vi "Autonomous Independent.vi"() -> ()   [LabVIEW 2015]
doc: "This VI is called when autonomous begins, and will automatically be terminated when autonomous ends. You can carry out timed or sensor driven robot movement independently without needing to return to the caller."
uses:
  <vilib>/Rock Robotics/WPI/Utilities/WPI_GetSetVariantRefNum.vi
  <vilib>/Rock Robotics/Network Tables/NT Read String.vi
  <vilib>/Rock Robotics/Network Tables/NT Write Number.vi
  <vilib>/addons/control/pid/pid.llb/PID (DBL).vi
  Robot Global Data.vi
  <vilib>/Rock Robotics/Network Tables/NT Write Numeric Array.vi
  <vilib>/addons/control/pid/NI_PID_pid.lvlib
  navX Library v2/navX Library v2.lvlib
panel:
  in  "Single Turn Gains":T1={"proportional gain (Kc)"=1.0, "integral time (Ti, min)"=0.01, "derivative time (Td, min)"=0.0} {"derivative time (Td, min)" format="%.3f"; "integral time (Ti, min)" format="%.3f"; "proportional gain (Kc)" format="%.3f"}
  in  "Yaw":T1={"proportional gain (Kc)"=1.0, "integral time (Ti, min)"=0.01, "derivative time (Td, min)"=0.0} {"derivative time (Td, min)" format="%.3f"; "integral time (Ti, min)" format="%.3f"; "proportional gain (Kc)" format="%.3f"}
  out "Right Motor Speed":dbl(graph)
  out "Left Motor Speed":dbl(graph)
  out "Right Motor":dbl(graph)
  out "Left Motor":dbl(graph)
  in  "Distance":dbl
  in  "Speed Gains 4":T1={"proportional gain (Kc)"=1.0, "integral time (Ti, min)"=0.01, "derivative time (Td, min)"=0.0} {"derivative time (Td, min)" format="%.3f"; "integral time (Ti, min)" format="%.3f"; "proportional gain (Kc)" format="%.3f"}
  out "E1 Dist 2":dbl
  out "E2 Dist 2":dbl
  out "nav X Yaw 2":dbl
  out "nav X Yaw":dbl
  out "E2 Dist":dbl
  out "E1 Dist":dbl
  in  "Yaw Gains":T1={"proportional gain (Kc)"=1.0, "integral time (Ti, min)"=0.01, "derivative time (Td, min)"=0.0} {"derivative time (Td, min)" format="%.3f"; "integral time (Ti, min)" format="%.3f"; "proportional gain (Kc)" format="%.3f"}
  # "Be sure to right-click and choose Data Operations>>Make Current Value default if you want to save the array values with the VI"
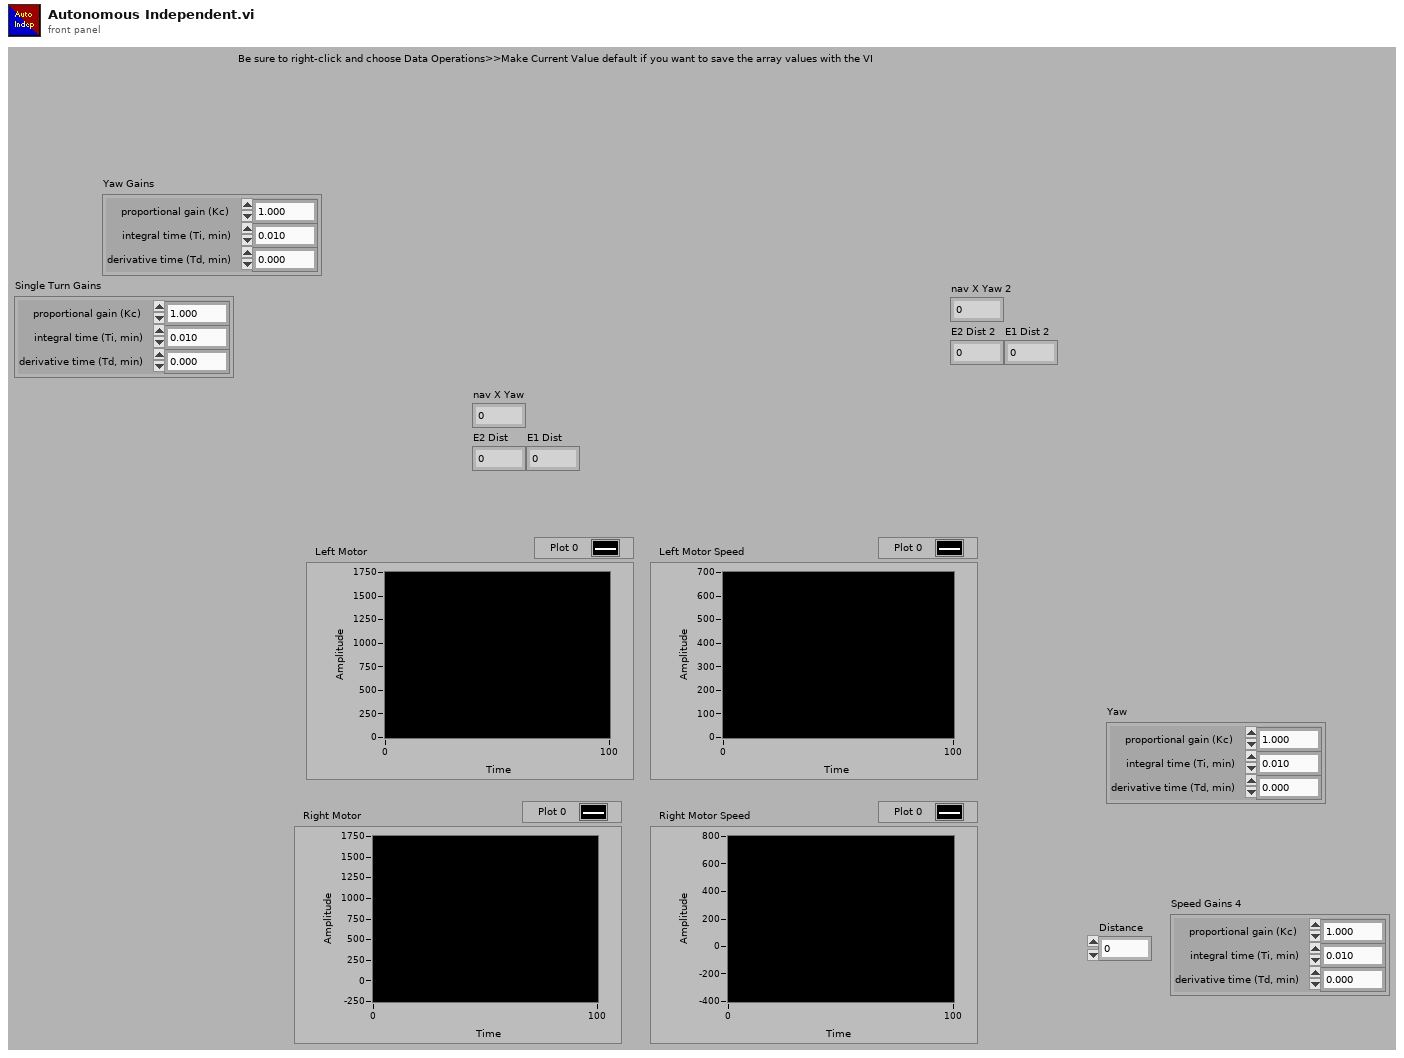
[diagram p1: front panel]
types:
  T1 = cluster{"proportional gain (Kc)":dbl, "integral time (Ti, min)":dbl, "derivative time (Td, min)":dbl}
  T2 = typedef "WPI_JoystickDevRef.ctl" = cluster{"Device":T3}
  T3 = typedef "WPI_JoystickDeviceEnum.ctl" = enum16{"USB 0", "USB 1", "USB 2", "USB 3", "USB 4", "USB 5"}
  T4 = typedef "navX Library v2.lvlib/Z900_navX_DeviceTypeDef.ctl" = cluster{"Interface":cluster{"Protocol":T5, "Update Rate (4Hz-60Hz)":u8, "navX Open TypeDef":variant}, "Notify Packet":refnum<notifier>, "Loop VI Refnum":refnum<vi>, "Ready to Close Occurrence Refnum":refnum<k4>}
  T5 = typedef "navX Library v2.lvlib/Z900_navX_ProtocolTypeDef.ctl" = enum16{"SERIAL", "I2C", "SPI"}
  T6 = typedef "WPI_EncoderDevRef.ctl" = cluster{"DevStatus":errorcluster, "EncoderIndex":T7, "CounterIndex":T8, "DistancePerCount":dbl, "Decoding Type":T9}
  T7 = typedef "FPGA_EncoderIdx.ctl" = enum8{"Enc 0", "Enc 1", "Enc 2", "Enc 3", "Enc 4", "Enc 5", "Enc 6", "Enc 7", "Invalid"}
  T8 = typedef "FPGA_CounterCtrSystemIndex.ctl" = enum8{"Ctr 0", "Ctr 1", "Ctr 2", "Ctr 3", "Ctr 4", "Ctr 5", "Ctr 6", "Ctr 7", "Invalid"}
  T9 = typedef "WPI_EncoderType.ctl" = enum16{"1x", "2x", "4x"}
  T10 = cluster{"Yaw":dbl, "Roll":dbl, "Pitch":dbl, "Heading":dbl, "Fused Heading":dbl}
  T11 = typedef "WPI_RobotDriveDevRef.ctl" = cluster{"DevStatus":errorcluster, "Motors[]":T12[], "Square Inputs":bool, "Max Output":dbl}
  T12 = typedef "WPI_MotorControlDeviceRef.ctl" = cluster{"DeviceStatus":errorcluster, "Type":T13, "PWM":cluster{"PWM Channel":T14, "DeadBand":T15}, "CAN":cluster{"Device Number":u8, "Control Mode":T16, "Semaphore":T17, "Max Vout":dbl, "TalonSRX Control Mode":T18}, "Invert":bool}
  T13 = typedef "WPI_MotorControlType.ctl" = enum16{"PWM", "CAN", "CANTalonSRX"}
  T14 = typedef "FPGA_DIOPWMChannel.ctl" = enum8{"PWM 0", "PWM 1", "PWM 2", "PWM 3", "PWM 4", "PWM 5", "PWM 6", "PWM 7", "PWM 8", "PWM 9", "PWM MXP 0", "PWM MXP 1", "PWM MXP 2", "PWM MXP 3", "PWM MXP 4", "PWM MXP 5", "PWM MXP 6", "PWM MXP 7", "PWM MXP 8", "PWM MXP 9", "Invalid"}
  T15 = typedef "WPI_PWMDeadband.ctl" = cluster{"Name":string, "maxPositivePwm":i32, "minPositivePwm":i32, "centerPwm":i32, "maxNegativePwm":i32, "minNegativePwm":i32, "angularRange":u16}
  T16 = typedef "WPI_CANJaguar_ControlMode.ctl" = enum8{"Percent VBus", "Current", "Speed", "Position", "Voltage"}
  T17 = typedef "Semaphore RefNum" = refnum<k1>
  T18 = typedef "WPI_CANTalonSRX_APIControlMode.ctl" = enum8{"Percent VBus", "Speed", "Position", "Slave", "Unchanged / Invalid", "Voltage Compensation", "Current", "Motion Profile"}
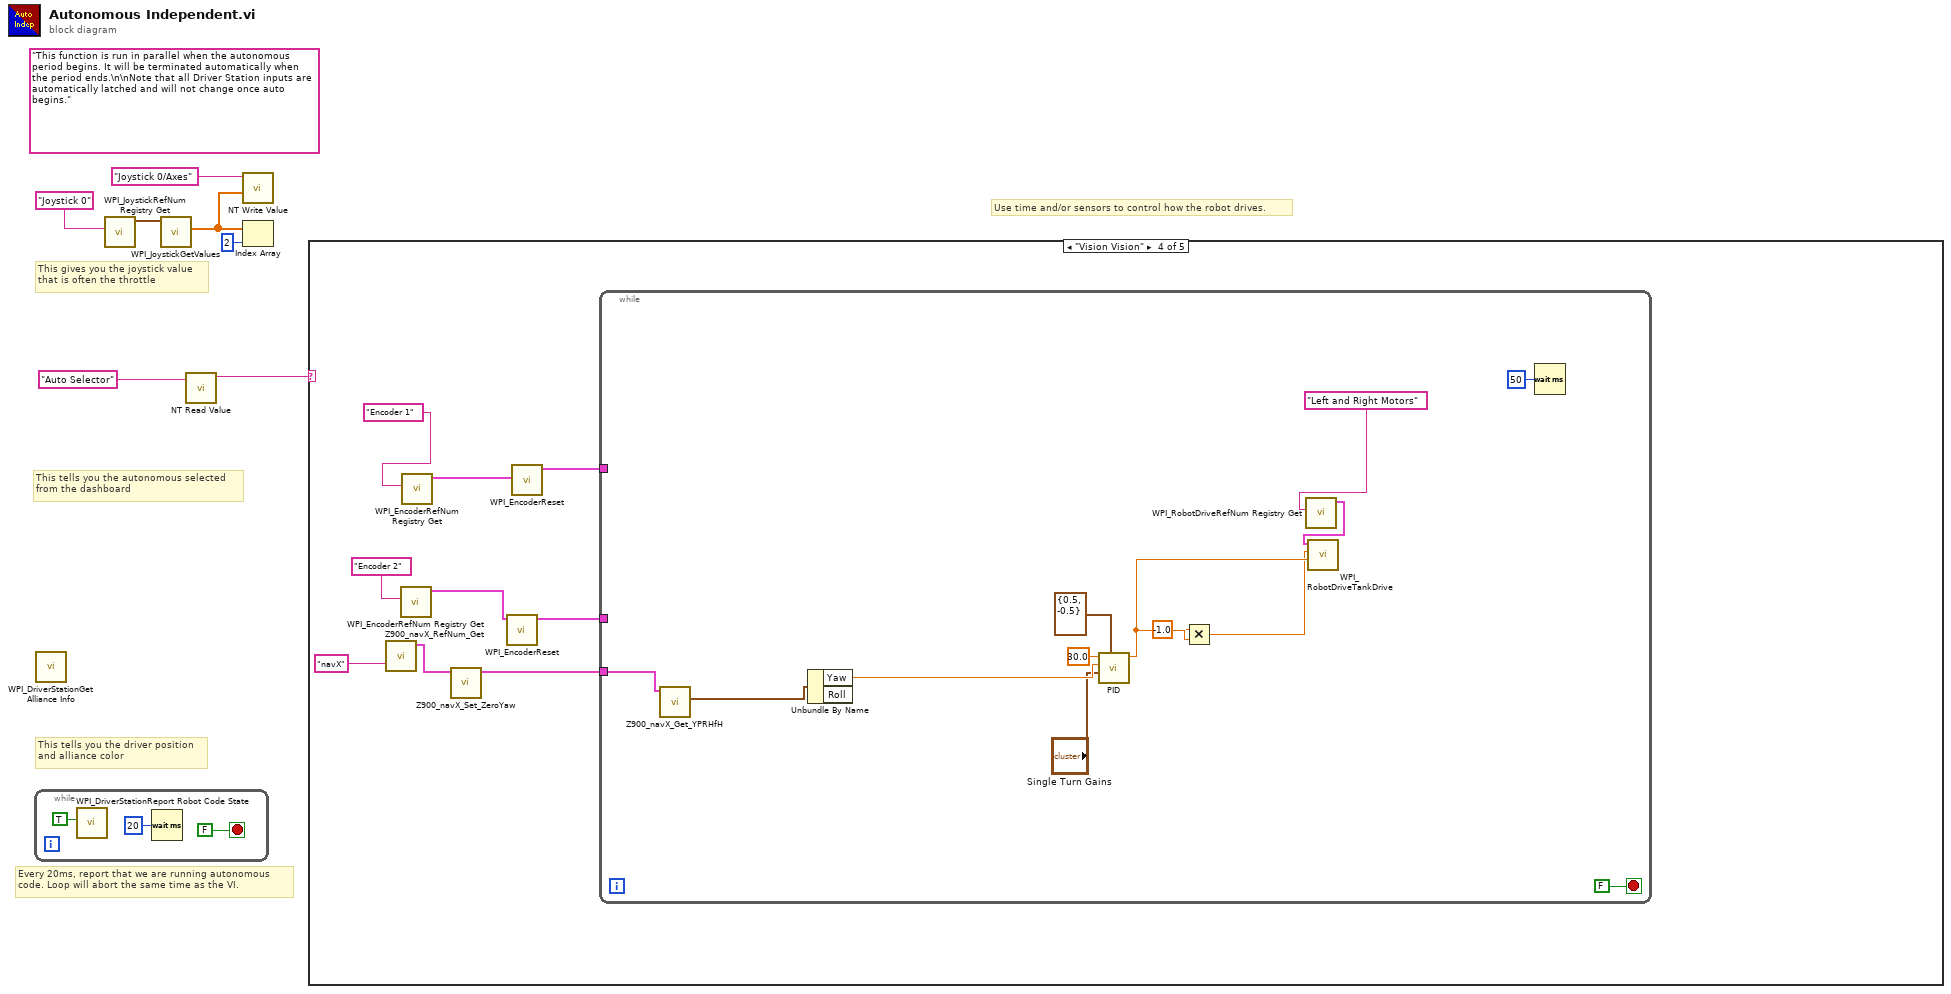
[diagram p0: block diagram]
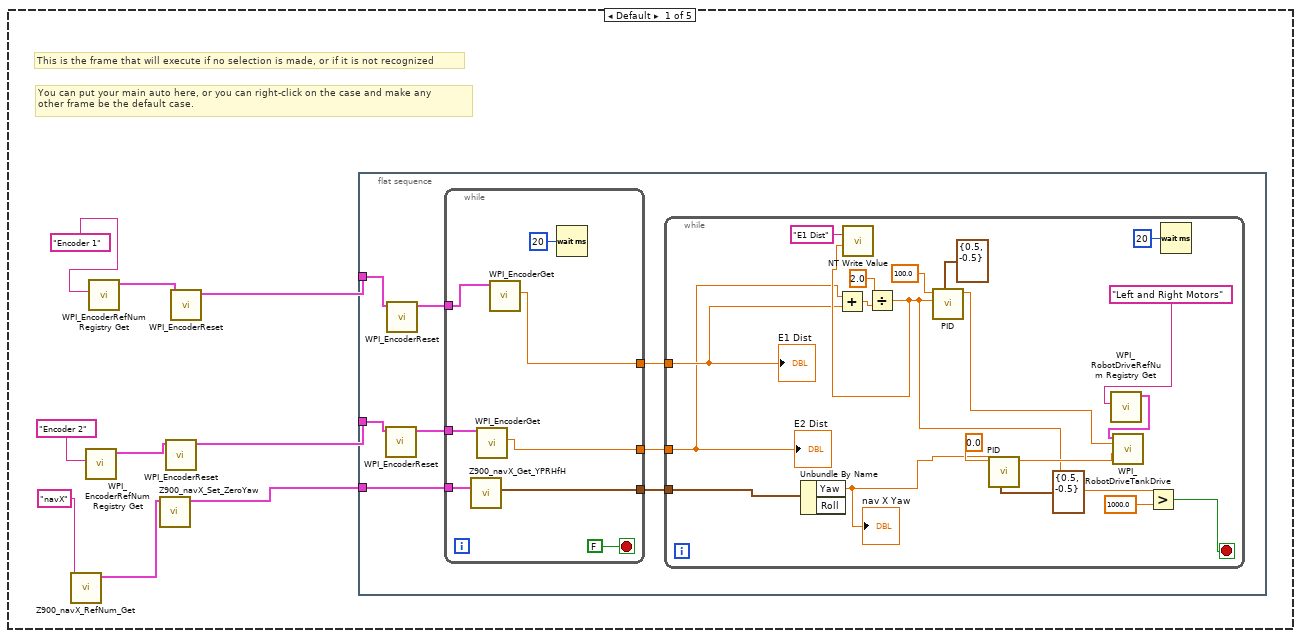
[diagram p2: hidden frame]
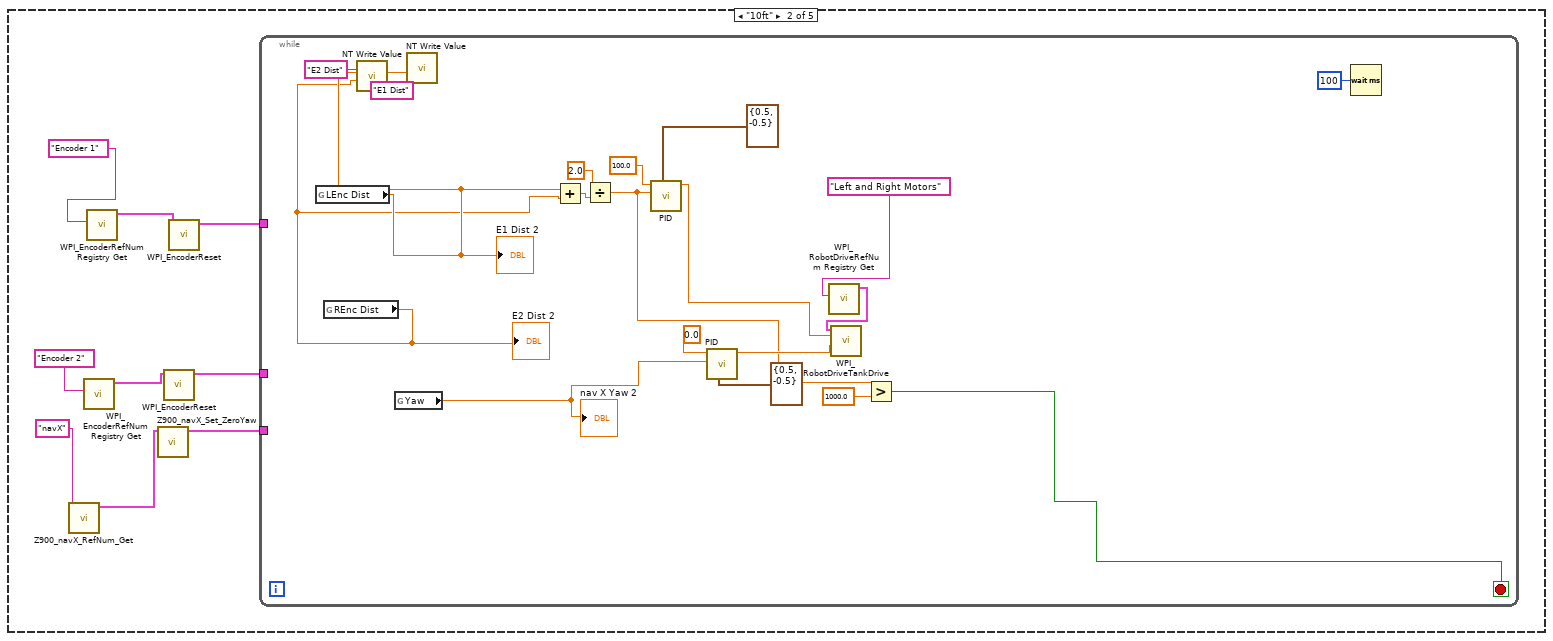
[diagram p3: hidden frame]
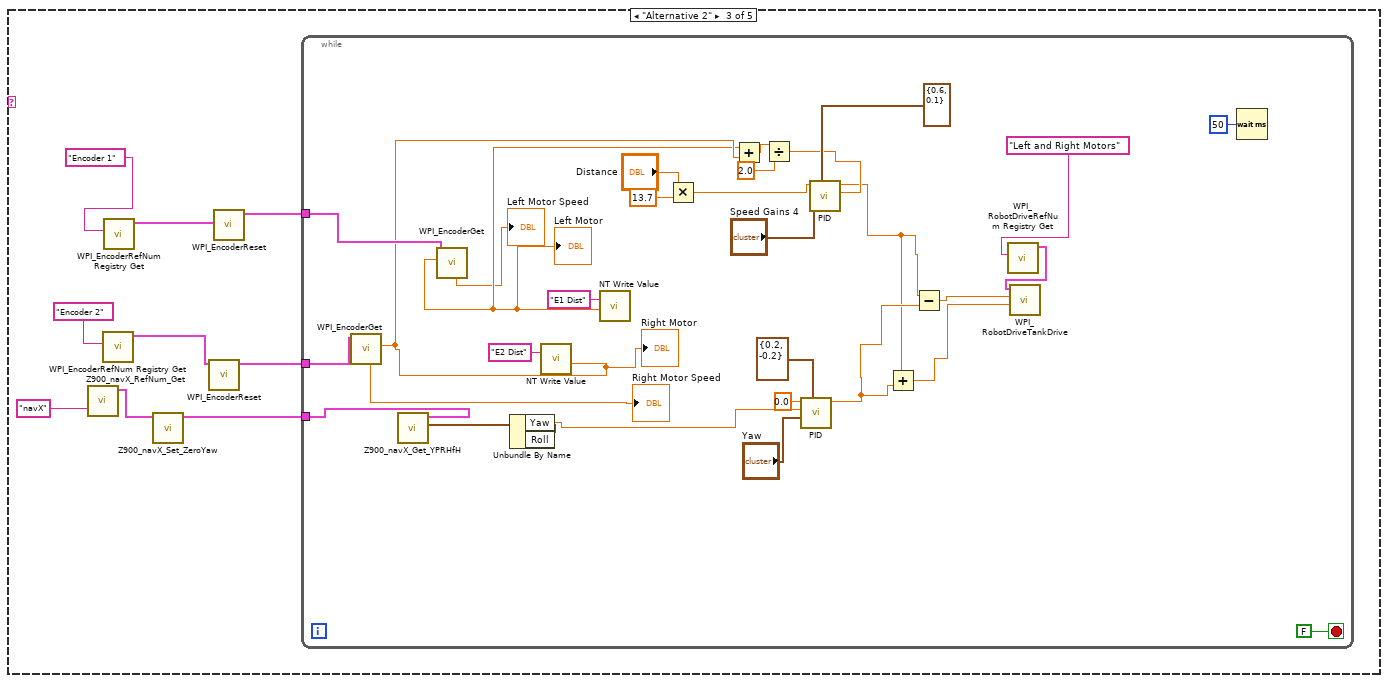
[diagram p4: hidden frame]
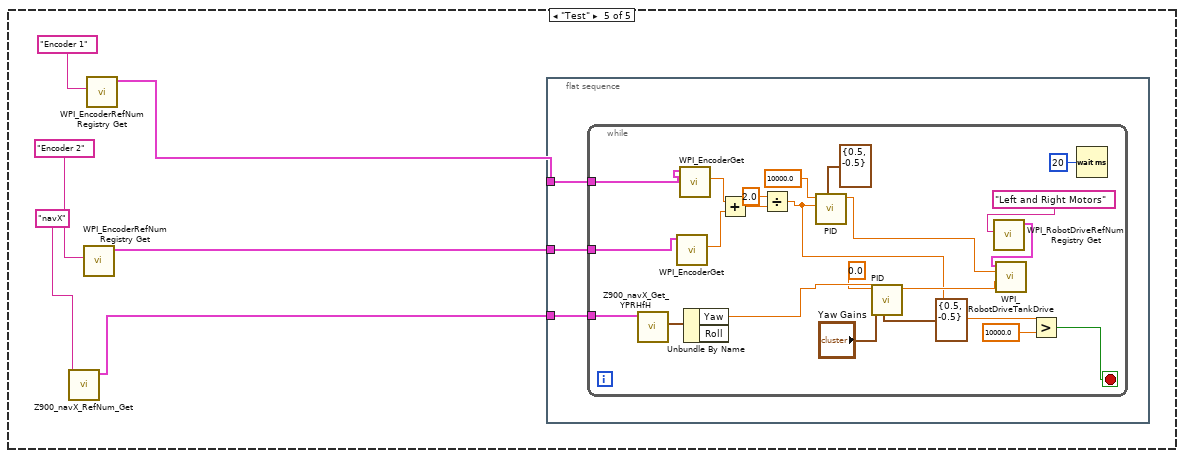
[diagram p5: hidden frame]
diagram:
  (unwired) "This function is run in parallel when the autonomous period begins. It will be terminated automatically when the period ends.\n\nNote that all Driver Station inputs are automatically latched and will not change once auto begins."
  # "This tells you the autonomous selected\nfrom the dashboard"
  # "Every 20ms, report that we are running autonomous\ncode. Loop will abort the same time as the VI."
  # "This gives you the joystick value\nthat is often the throttle"
  # "Use time and/or sensors to control how the robot drives."
  # "This tells you the driver position\nand alliance color"
  n1 = while {
    stop <- FALSE stop-if-true
    n2 = call <vilib>:"WPI_DriverStationReport Robot Code State.vi"("Autonomous"=TRUE) -> ()  [unwired: 10 in, 1 out]
    n3 = Wait (ms)(milliseconds to wait=u32 20) -> ()  [unwired: 1 out]
  }
  n4 = call <vilib>:"WPI_DriverStationGet Alliance Info.vi"() -> ()  [unwired: 12 out]
  n5 = call <vilib>:"WPI_JoystickRefNum Registry Get.vi"("refnum name"="Joystick 0") -> ("JoystickDevRef"=w6:T2)  [unwired: 1 in, 9 out]
  n6 = call <vilib>:"WPI_JoystickGetValues.vi"("JoystickDevRef"=w6) -> ("Axes"=w2:dbl[])  [unwired: 6 in, 4 out]
  n7 = call-poly <vilib>:"NT Read Value.vi"("Name"="Auto Selector") -> ("String"=w3:string)  [unwired: 9 in, 1 out]
  n8 = call-poly <vilib>:"NT Write Value.vi"("Numeric Array"=w2, "Name"="Joystick 0/Axes") -> ()  [unwired: 9 in, 1 out]
  n9 = Index Array(array=w2, index=2) -> ()  [unwired: 1 out]
  n10 = case shown="\"Vision Vision\"" w3 {
    frame Default {
      # "You can put your main auto here, or you can right-click on the case and make any\nother frame be the default case."
      # "This is the frame that will execute if no selection is made, or if it is not recognized"
      n11 = call "Z900_navX_RefNum_Get.vi"("refnum name"="navX") -> ("navX Device"=w13:T4)  [unwired: 9 in, 1 out]
      n12 = call <vilib>:"WPI_EncoderRefNum Registry Get.vi"("refnum name"="Encoder 2") -> ("EncoderDevRef"=w15:T6)  [unwired: 9 in, 1 out]
      n13 = call <vilib>:"WPI_EncoderRefNum Registry Get.vi"("refnum name"="Encoder 1") -> ("EncoderDevRef"=w17:T6)  [unwired: 9 in, 1 out]
      n14 = call "Z900_navX_Set_ZeroYaw.vi"("navX Device"=w13) -> ("navX Device"=w12:T4)  [unwired: 9 in, 1 out]
      n15 = call <vilib>:"WPI_EncoderReset.vi"("EncoderDevRef"=w15) -> ("EncoderDevRef"=w14:T6)  [unwired: 9 in, 1 out]
      n16 = call <vilib>:"WPI_EncoderReset.vi"("EncoderDevRef"=w17) -> ("EncoderDevRef"=w16:T6)  [unwired: 9 in, 1 out]
      n17 = flat-sequence {
        tunnel: w16 -> [w27]
        tunnel: w14 -> [w26]
        tunnel: w12 -> [w25]
        frame #0 {
          n18 = call <vilib>:"WPI_EncoderReset.vi"("EncoderDevRef"=w26) -> ("EncoderDevRef"=w24:T6)  [unwired: 9 in, 1 out]
          n19 = call <vilib>:"WPI_EncoderReset.vi"("EncoderDevRef"=w27) -> ("EncoderDevRef"=w23:T6)  [unwired: 9 in, 1 out]
          n20 = while {
            tunnel: w25 -> [w32]
            tunnel: w24 -> [w33]
            tunnel: w23 -> [w34]
            tunnel: [w31] -> w22
            tunnel: [w30] -> w21
            tunnel: [w29] -> w20
            stop <- FALSE stop-if-true
            n21 = call "Z900_navX_Get_YPRHfH.vi"("navX Device"=w32) -> ("YRPHfH"=w31:T10)  [unwired: 7 in, 3 out]
            n22 = call <vilib>:"WPI_EncoderGet.vi"("EncoderDevRef"=w33) -> ("Distance"=w30:dbl)  [unwired: 5 in, 5 out]
            n23 = call <vilib>:"WPI_EncoderGet.vi"("EncoderDevRef"=w34) -> ("Distance"=w29:dbl)  [unwired: 5 in, 5 out]
            n24 = Wait (ms)(milliseconds to wait=u32 20) -> ()  [unwired: 1 out]
          }
          n25 = while {
            tunnel: w22 -> [w39]
            tunnel: w21 -> [w37]
            tunnel: w20 -> [w38]
            stop <- w43 stop-if-true
            n26 = Unbundle By Name(w39) -> ("Yaw"=w40:dbl)  [unwired: 1 out]
            "nav X Yaw" <- w40
            n27 = Add(x=w37, y=w38) -> (x+y=w54:dbl)
            n28 = Divide(x=2.0, y=w54) -> (x/y=w42:dbl)
            n29 = call-poly <vilib>:"NT Write Value.vi"("Numeric"=w42, "Name"="E1 Dist") -> ()  [unwired: 9 in, 1 out]
            n30 = call-poly <vilib>:"PID.vi"("output range"=cluster{"output high":dbl, "output low":dbl} {"output high"=0.5, "output low"=-0.5}, "process variable"=w42, "setpoint"=100.0) -> ("output"=w47:dbl)  [unwired: 7 in, 1 out]
            n31 = call-poly <vilib>:"PID.vi"("output range"=cluster{"output high":dbl, "output low":dbl} {"output high"=0.5, "output low"=-0.5}, "process variable"=w40, "setpoint"=0.0) -> ("output"=w46:dbl)  [unwired: 7 in, 1 out]
            n32 = call <vilib>:"WPI_RobotDriveRefNum Registry Get.vi"("refnum name"="Left and Right Motors") -> ("RobotDriveDevRef"=w49:T11)  [unwired: 9 in, 1 out]
            n33 = call <vilib>:"WPI_RobotDriveTankDrive.vi"("Right axis value"=w46, "Left axis value"=w47, "RobotDriveDevRef"=w49) -> ()  [unwired: 6 in, 3 out]
            n34 = Greater?(x=w42, y=1000.0) -> (0:w43:bool)
            n35 = Wait (ms)(milliseconds to wait=u32 20) -> ()  [unwired: 1 out]
            "E2 Dist" <- w37
            "E1 Dist" <- w38
          }
        }
      }
    }
    frame "10ft" {
      n36 = call "Z900_navX_RefNum_Get.vi"("refnum name"="navX") -> ("navX Device"=w57:T4)  [unwired: 9 in, 1 out]
      n37 = call <vilib>:"WPI_EncoderRefNum Registry Get.vi"("refnum name"="Encoder 2") -> ("EncoderDevRef"=w59:T6)  [unwired: 9 in, 1 out]
      n38 = call <vilib>:"WPI_EncoderRefNum Registry Get.vi"("refnum name"="Encoder 1") -> ("EncoderDevRef"=w61:T6)  [unwired: 9 in, 1 out]
      n39 = call "Z900_navX_Set_ZeroYaw.vi"("navX Device"=w57) -> ("navX Device"=w56:T4)  [unwired: 9 in, 1 out]
      n40 = call <vilib>:"WPI_EncoderReset.vi"("EncoderDevRef"=w59) -> ("EncoderDevRef"=w58:T6)  [unwired: 9 in, 1 out]
      n41 = call <vilib>:"WPI_EncoderReset.vi"("EncoderDevRef"=w61) -> ("EncoderDevRef"=w60:T6)  [unwired: 9 in, 1 out]
      n42 = while {
        tunnel: w60 -> [_]
        tunnel: w58 -> [_]
        tunnel: w56 -> [_]
        stop <- w64 stop-if-true
        n43 = global read "Robot Global Data.vi" "LEnc Dist"() -> (w67:dbl)
        "E1 Dist 2" <- w67
        n44 = global read "Robot Global Data.vi" "REnc Dist"() -> (w66:dbl)
        "E2 Dist 2" <- w66
        n45 = call-poly <vilib>:"NT Write Value.vi"("Numeric"=w66, "Name"="E2 Dist") -> ()  [unwired: 9 in, 1 out]
        n46 = global read "Robot Global Data.vi" "Yaw"() -> (w65:dbl)
        "nav X Yaw 2" <- w65
        n47 = call-poly <vilib>:"NT Write Value.vi"("Numeric"=w67, "Name"="E1 Dist") -> ()  [unwired: 9 in, 1 out]
        n48 = Add(x=w67, y=w66) -> (x+y=w81:dbl)
        n49 = Divide(x=2.0, y=w81) -> (x/y=w71:dbl)
        n50 = call-poly <vilib>:"PID.vi"("output range"=cluster{"output high":dbl, "output low":dbl} {"output high"=0.5, "output low"=-0.5}, "process variable"=w71, "setpoint"=100.0) -> ("output"=w75:dbl)  [unwired: 7 in, 1 out]
        n51 = call-poly <vilib>:"PID.vi"("output range"=cluster{"output high":dbl, "output low":dbl} {"output high"=0.5, "output low"=-0.5}, "process variable"=w65, "setpoint"=0.0) -> ("output"=w74:dbl)  [unwired: 7 in, 1 out]
        n52 = call <vilib>:"WPI_RobotDriveRefNum Registry Get.vi"("refnum name"="Left and Right Motors") -> ("RobotDriveDevRef"=w77:T11)  [unwired: 9 in, 1 out]
        n53 = call <vilib>:"WPI_RobotDriveTankDrive.vi"("Right axis value"=w74, "Left axis value"=w75, "RobotDriveDevRef"=w77) -> ()  [unwired: 6 in, 3 out]
        n54 = Greater?(x=w71, y=1000.0) -> (0:w64:bool)
        n55 = Wait (ms)(milliseconds to wait=u32 100) -> ()  [unwired: 1 out]
      }
    }
    frame "Alternative 2" {
      n56 = call "Z900_navX_RefNum_Get.vi"("refnum name"="navX") -> ("navX Device"=w84:T4)  [unwired: 9 in, 1 out]
      n57 = call <vilib>:"WPI_EncoderRefNum Registry Get.vi"("refnum name"="Encoder 2") -> ("EncoderDevRef"=w86:T6)  [unwired: 9 in, 1 out]
      n58 = call <vilib>:"WPI_EncoderRefNum Registry Get.vi"("refnum name"="Encoder 1") -> ("EncoderDevRef"=w88:T6)  [unwired: 9 in, 1 out]
      n59 = call "Z900_navX_Set_ZeroYaw.vi"("navX Device"=w84) -> ("navX Device"=w83:T4)  [unwired: 9 in, 1 out]
      n60 = call <vilib>:"WPI_EncoderReset.vi"("EncoderDevRef"=w86) -> ("EncoderDevRef"=w85:T6)  [unwired: 9 in, 1 out]
      n61 = call <vilib>:"WPI_EncoderReset.vi"("EncoderDevRef"=w88) -> ("EncoderDevRef"=w87:T6)  [unwired: 9 in, 1 out]
      n62 = while {
        tunnel: w87 -> [w114]
        tunnel: w85 -> [w113]
        tunnel: w83 -> [w112]
        stop <- FALSE stop-if-true
        n63 = call <vilib>:"WPI_EncoderGet.vi"("EncoderDevRef"=w113) -> ("Distance"=w103:dbl, "Rate"=→"Right Motor Speed":dbl)  [unwired: 5 in, 4 out]
        "Right Motor" <- w103
        n64 = call "Z900_navX_Get_YPRHfH.vi"("navX Device"=w112) -> ("YRPHfH"=w115:T10)  [unwired: 7 in, 3 out]
        n65 = call <vilib>:"WPI_EncoderGet.vi"("EncoderDevRef"=w114) -> ("Distance"=w102:dbl, "Rate"=→"Left Motor Speed":dbl)  [unwired: 5 in, 4 out]
        "Left Motor" <- w102
        n66 = Unbundle By Name(w115) -> ("Yaw"=w99:dbl)  [unwired: 1 out]
        n67 = call-poly <vilib>:"NT Write Value.vi"("Numeric"=w103, "Name"="E2 Dist") -> ()  [unwired: 9 in, 1 out]
        n68 = call-poly <vilib>:"NT Write Value.vi"("Numeric"=w102, "Name"="E1 Dist") -> ()  [unwired: 9 in, 1 out]
        n69 = Multiply(x="Distance", y=13.7) -> (x*y=w104:dbl)
        n70 = Add(x=w102, y=w103) -> (x+y=w109:dbl)
        n71 = Divide(x=w109, y=2.0) -> (x/y=w107:dbl)
        n72 = call-poly <vilib>:"PID.vi"("output range"=cluster{"output high":dbl, "output low":dbl} {"output high"=0.2, "output low"=-0.2}, "PID gains"="Yaw", "process variable"=w99, "setpoint"=0.0) -> ("output"=w97:dbl)  [unwired: 6 in, 1 out]
        n73 = call-poly <vilib>:"PID.vi"("output range"=cluster{"output high":dbl, "output low":dbl} {"output high"=0.6, "output low"=0.1}, "PID gains"="Speed Gains 4", "process variable"=w107, "setpoint"=w104) -> ("output"=w94:dbl)  [unwired: 6 in, 1 out]
        n74 = Add(x=w94, y=w97) -> (x+y=w96:dbl)
        n75 = Subtract(x=w94, y=w97) -> (x-y=w95:dbl)
        n76 = call <vilib>:"WPI_RobotDriveRefNum Registry Get.vi"("refnum name"="Left and Right Motors") -> ("RobotDriveDevRef"=w117:T11)  [unwired: 9 in, 1 out]
        n77 = call <vilib>:"WPI_RobotDriveTankDrive.vi"("Right axis value"=w96, "Left axis value"=w95, "RobotDriveDevRef"=w117) -> ()  [unwired: 6 in, 3 out]
        n78 = Wait (ms)(milliseconds to wait=u32 50) -> ()  [unwired: 1 out]
      }
    }
    frame "Vision Vision" {
      n79 = call "Z900_navX_RefNum_Get.vi"("refnum name"="navX") -> ("navX Device"=w123:T4)  [unwired: 9 in, 1 out]
      n80 = call <vilib>:"WPI_EncoderRefNum Registry Get.vi"("refnum name"="Encoder 2") -> ("EncoderDevRef"=w125:T6)  [unwired: 9 in, 1 out]
      n81 = call <vilib>:"WPI_EncoderRefNum Registry Get.vi"("refnum name"="Encoder 1") -> ("EncoderDevRef"=w127:T6)  [unwired: 9 in, 1 out]
      n82 = call "Z900_navX_Set_ZeroYaw.vi"("navX Device"=w123) -> ("navX Device"=w122:T4)  [unwired: 9 in, 1 out]
      n83 = call <vilib>:"WPI_EncoderReset.vi"("EncoderDevRef"=w125) -> ("EncoderDevRef"=w124:T6)  [unwired: 9 in, 1 out]
      n84 = call <vilib>:"WPI_EncoderReset.vi"("EncoderDevRef"=w127) -> ("EncoderDevRef"=w126:T6)  [unwired: 9 in, 1 out]
      n85 = while {
        tunnel: w126 -> [_]
        tunnel: w124 -> [_]
        tunnel: w122 -> [w137]
        stop <- FALSE stop-if-true
        n86 = call "Z900_navX_Get_YPRHfH.vi"("navX Device"=w137) -> ("YRPHfH"=w136:T10)  [unwired: 7 in, 3 out]
        n87 = Unbundle By Name(w136) -> ("Yaw"=w135:dbl)  [unwired: 1 out]
        n88 = call-poly <vilib>:"PID.vi"("output range"=cluster{"output high":dbl, "output low":dbl} {"output high"=0.5, "output low"=-0.5}, "PID gains"="Single Turn Gains", "process variable"=w135, "setpoint"=30.0) -> ("output"=w133:dbl)  [unwired: 6 in, 1 out]
        n89 = Multiply(x=-1.0, y=w133) -> (x*y=w131:dbl)
        n90 = call <vilib>:"WPI_RobotDriveRefNum Registry Get.vi"("refnum name"="Left and Right Motors") -> ("RobotDriveDevRef"=w142:T11)  [unwired: 9 in, 1 out]
        n91 = call <vilib>:"WPI_RobotDriveTankDrive.vi"("Right axis value"=w133, "Left axis value"=w131, "RobotDriveDevRef"=w142) -> ()  [unwired: 6 in, 3 out]
        n92 = Wait (ms)(milliseconds to wait=u32 50) -> ()  [unwired: 1 out]
      }
    }
    frame "Test" {
      n93 = call "Z900_navX_RefNum_Get.vi"("refnum name"="navX") -> ("navX Device"=w144:T4)  [unwired: 9 in, 1 out]
      n94 = call <vilib>:"WPI_EncoderRefNum Registry Get.vi"("refnum name"="Encoder 2") -> ("EncoderDevRef"=w145:T6)  [unwired: 9 in, 1 out]
      n95 = call <vilib>:"WPI_EncoderRefNum Registry Get.vi"("refnum name"="Encoder 1") -> ("EncoderDevRef"=w146:T6)  [unwired: 9 in, 1 out]
      n96 = flat-sequence {
        tunnel: w146 -> [w152]
        tunnel: w145 -> [w151]
        tunnel: w144 -> [w150]
        frame #0 {
          n97 = while {
            tunnel: w152 -> [w173]
            tunnel: w151 -> [w172]
            tunnel: w150 -> [w163]
            stop <- w153 stop-if-true
            n98 = call "Z900_navX_Get_YPRHfH.vi"("navX Device"=w163) -> ("YRPHfH"=w174:T10)  [unwired: 7 in, 3 out]
            n99 = call <vilib>:"WPI_EncoderGet.vi"("EncoderDevRef"=w172) -> ("Distance"=w169:dbl)  [unwired: 5 in, 5 out]
            n100 = call <vilib>:"WPI_EncoderGet.vi"("EncoderDevRef"=w173) -> ("Distance"=w170:dbl)  [unwired: 5 in, 5 out]
            n101 = Unbundle By Name(w174) -> ("Yaw"=w165:dbl)  [unwired: 1 out]
            n102 = Add(x=w170, y=w169) -> (x+y=w168:dbl)
            n103 = Divide(x=2.0, y=w168) -> (x/y=w155:dbl)
            n104 = call-poly <vilib>:"PID.vi"("output range"=cluster{"output high":dbl, "output low":dbl} {"output high"=0.5, "output low"=-0.5}, "process variable"=w155, "setpoint"=10000.0) -> ("output"=w159:dbl)  [unwired: 7 in, 1 out]
            n105 = call-poly <vilib>:"PID.vi"("output range"=cluster{"output high":dbl, "output low":dbl} {"output high"=0.5, "output low"=-0.5}, "PID gains"="Yaw Gains", "process variable"=w165, "setpoint"=0.0) -> ("output"=w158:dbl)  [unwired: 6 in, 1 out]
            n106 = call <vilib>:"WPI_RobotDriveRefNum Registry Get.vi"("refnum name"="Left and Right Motors") -> ("RobotDriveDevRef"=w161:T11)  [unwired: 9 in, 1 out]
            n107 = call <vilib>:"WPI_RobotDriveTankDrive.vi"("Right axis value"=w158, "Left axis value"=w159, "RobotDriveDevRef"=w161) -> ()  [unwired: 6 in, 3 out]
            n108 = Greater?(x=w155, y=10000.0) -> (0:w153:bool)
            n109 = Wait (ms)(milliseconds to wait=u32 20) -> ()  [unwired: 1 out]
          }
        }
      }
    }
  }
